vi "Initiate.vi"(8 "error in (no error)":errorcluster) -> (0 "error out":errorcluster, 3 "Simulation Interface out":refnum<class "Simulation Interface.lvclass">)   [LabVIEW 2012, in "Simulation Interface.lvclass"]
uses:
  Simulation Interface.lvclass
  Car Wash Controller/Car Wash Controller.lvclass
  Entry Console/Entry Console.lvclass
  Vehicle Position Simulation/Vehicle Position Simulation.lvclass
  Wash Display Console/Wash Display Console.lvclass
  Database/Database.lvclass
  Error Handler/Error Handler.lvclass
  Error Handler/EH Action.ctl
  Thread/Thread.lvclass
  Database/Database Action.ctl
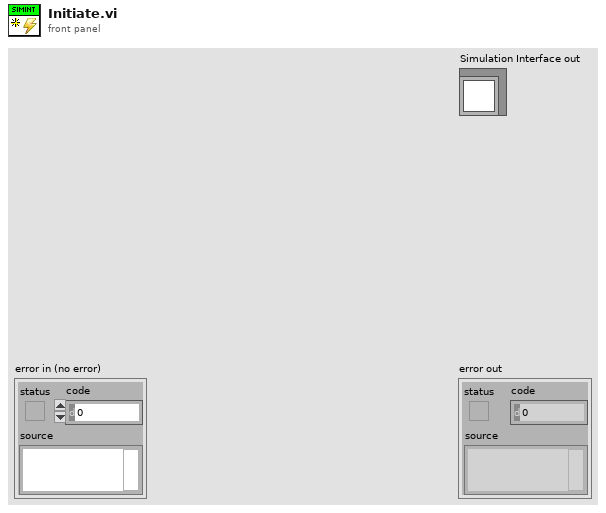
[diagram p1: front panel]
types:
  T1 = typedef "Architecture.lvlib/Error Handler.lvclass/EH Action.ctl" = enum16{"Define Threads", "Close", "System Error", "Wash Cycle Error", "Minor Error", "Initialize"}
  T2 = typedef "Architecture.lvlib/Database.lvclass/Database Action.ctl" = enum16{"Update Data Record", "Insert New Data Record", "Query Timing Data", "Read Records", "Initialize"}
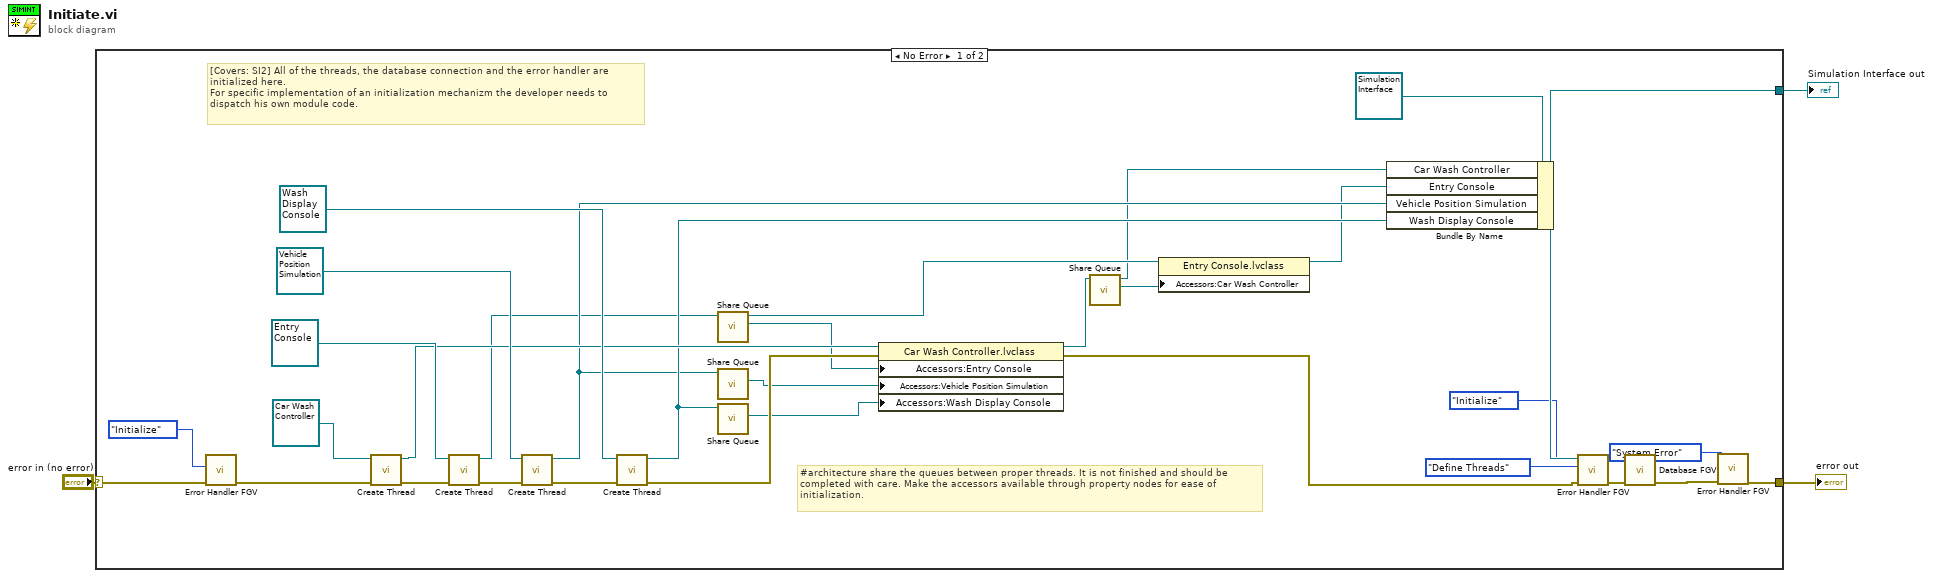
[diagram p0: block diagram]
diagram:
  n1 = case shown="No Error" "error in (no error)" {
    selector: "error in (no error)" -> [w27 w36]
    tunnel: [w6 w36] -> w2
    tunnel: [w22 _] -> w1
    frame No Error {
      # "#architecture share the queues between proper threads. It is not finished and should be \ncompleted with care. Make the accessors available through property nodes for ease of\ninitialization."
      # "[Covers: SI2] All of the threads, the database connection and the error handler are\ninitialized here.\nFor specific implementation of an initialization mechanizm the developer needs to\ndispatch his own module code."
      n2 = call "Error Handler FGV.vi"("error in (no error)"=w27, "Action"=EH_Action."Initialize") -> ("error out"=w26:errorcluster)  [unwired: 9 in]
      n3 = call-dynamic "Create Thread.vi"("error in (no error)"=w26, "Thread in"=refnum<class "Car Wash Controller.lvclass"> refnum ("Car Wash Controller.lvlib:Car Wash Controller.lvclass")) -> ("error out"=w34:errorcluster, "Thread out"=w21:refnum<class "Car Wash Controller.lvclass">)  [unwired: 8 in]
      n4 = call-dynamic "Create Thread.vi"("error in (no error)"=w34, "Thread in"=refnum<class "Entry Console.lvclass"> refnum ("Entry Console.lvlib:Entry Console.lvclass")) -> ("error out"=w33:errorcluster, "Thread out"=w13:refnum<class "Entry Console.lvclass">)  [unwired: 8 in]
      n5 = call-dynamic "Create Thread.vi"("error in (no error)"=w33, "Thread in"=refnum<class "Vehicle Position Simulation.lvclass"> refnum ("Vehicle Position Simulation.lvlib:Vehicle Position Simulation.lvclass")) -> ("error out"=w32:errorcluster, "Thread out"=w15:refnum<class "Vehicle Position Simulation.lvclass">)  [unwired: 8 in]
      n6 = call-dynamic "Create Thread.vi"("error in (no error)"=w32, "Thread in"=refnum<class "Wash Display Console.lvclass"> refnum ("Wash Display Console.lvlib:Wash Display Console.lvclass")) -> ("error out"=w20:errorcluster, "Thread out"=w18:refnum<class "Wash Display Console.lvclass">)  [unwired: 8 in]
      n7 = call "Share Queue.vi"("Thread in"=w13) -> ("Architecture.lvlib:Queue.lvclass"=w14:refnum<class "Queue.lvclass">, "Thread out"=w12:refnum<class "Entry Console.lvclass">)  [unwired: 8 in, 1 out]
      n8 = call "Share Queue.vi"("Thread in"=w15) -> ("Architecture.lvlib:Queue.lvclass"=w16:refnum<class "Queue.lvclass">)  [unwired: 8 in, 2 out]
      n9 = call "Share Queue.vi"("Thread in"=w18) -> ("Architecture.lvlib:Queue.lvclass"=w17:refnum<class "Queue.lvclass">)  [unwired: 8 in, 2 out]
      n10 = property class="Car Wash Controller.lvclass"(reference=w21, error in=w20, "Accessors:Entry Console"=w14, "Accessors:Vehicle Position Simulation"=w16, "Accessors:Wash Display Console"=w17) -> (reference out=w11:refnum<class "Car Wash Controller.lvclass">, error out=w19:errorcluster)
      n11 = call "Share Queue.vi"("Thread in"=w11) -> ("Architecture.lvlib:Queue.lvclass"=w10:refnum<class "Queue.lvclass">, "Thread out"=w9:refnum<class "Car Wash Controller.lvclass">)  [unwired: 8 in, 1 out]
      n12 = property class="Entry Console.lvclass"(reference=w12, "Accessors:Car Wash Controller"=w10) -> (reference out=w8:refnum<class "Entry Console.lvclass">)  [unwired: 1 in, 1 out]
      n13 = Bundle By Name(cluster=refnum<class "Simulation Interface.lvclass"> refnum ("Simulation Interface.lvclass"), "Car Wash Controller"=w9, "Entry Console"=w8, "Vehicle Position Simulation"=w15, "Wash Display Console"=w18) -> (w22:refnum<class "Simulation Interface.lvclass">)
      n14 = call "Error Handler FGV.vi"("error in (no error)"=w19, "Action"=EH_Action."Define Threads", "Application to EH"=w22) -> ("error out"=w23:errorcluster)  [unwired: 8 in]
      n15 = call "Database FGV.vi"("error in (no error)"=w23, "Database Action"=Database_Action."Initialize") -> ("error out"=w7:errorcluster)  [unwired: 7 in, 2 out]
      n16 = call "Error Handler FGV.vi"("error in (no error)"=w7, "Action"=EH_Action."System Error") -> ("error out"=w6:errorcluster)  [unwired: 9 in]
    }
    frame Error {
    }
  }
  "error out" <- w2
  "Simulation Interface out" <- w1
